vi "Do.vi"(8 "error in (no error)":errorcluster, 10 "Actor in":refnum<class "Actor.lvclass">, 11 "Configure Arbitrary Sequence [SEQ] Msg":refnum<class "Configure Arbitrary Sequence [SEQ] Msg.lvclass">) -> (0 "error out":errorcluster, 2 "Actor out":refnum<class "Actor.lvclass">)   [LabVIEW 2014, in "CS++Fgen.lvlib" / "Configure Arbitrary Sequence [SEQ] Msg.lvclass"]
doc: "This VI delivers the message to the actor by calling the appropriate method(s) on the actor."
uses:
  Configure Arbitrary Sequence [SEQ] Msg.lvclass
  <vilib>/ActorFramework/Actor/Actor.lvclass
  CS++Fgen/CS++Fgen.lvclass
  Configure Arbitrary Sequence [SEQ].ctl
  CSPP_Core/Actors/CS++PVMonitor Messages/CS++PVUpdate Msg/CS++PVUpdate Msg.lvclass/CS++PVUpdate Msg.ctl
  CSPP_Core/Classes/CS++ProcessVariables/ProcessVariable/PV.lvclass/PV.ctl
  Configure Arbitrary Sequence [SEQ] Msg.lvclass/Configure Arbitrary Sequence [SEQ] Msg.ctl
  CSPP_Core/Classes/CS++ProcessVariables/ProcessVariable/PV.lvclass
  CSPP_Core/Actors/CS++PVMonitor Messages/CS++PVUpdate Msg/CS++PVUpdate Msg.lvclass
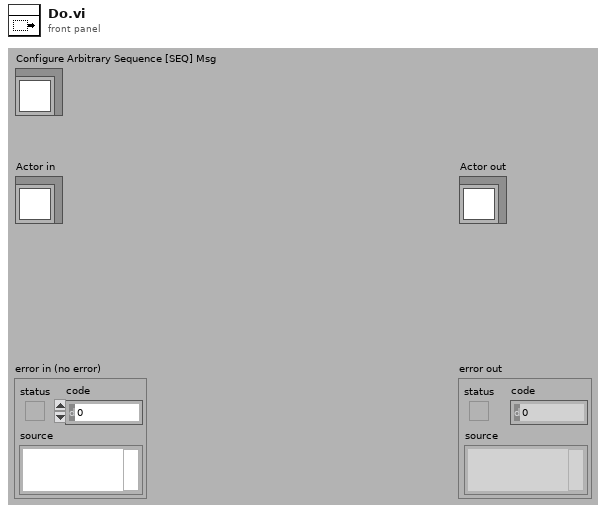
[diagram p1: front panel]
types:
  T1 = typedef "CS++Fgen.lvlib/Configure Arbitrary Sequence [SEQ] Msg.lvclass/Configure Arbitrary Sequence [SEQ].ctl" = cluster{"channel name (\"CHANNEL1\")":string, "offset (0.00 V)":dbl[unit], "gain (1.00)":dbl, "sequence handle (0)":i32}
  T2 = cluster{"channel name (\"CHANNEL1\")":string, "offset (0.00 V)":dbl[unit], "gain (1.00)":dbl, "sequence handle (0)":i32}
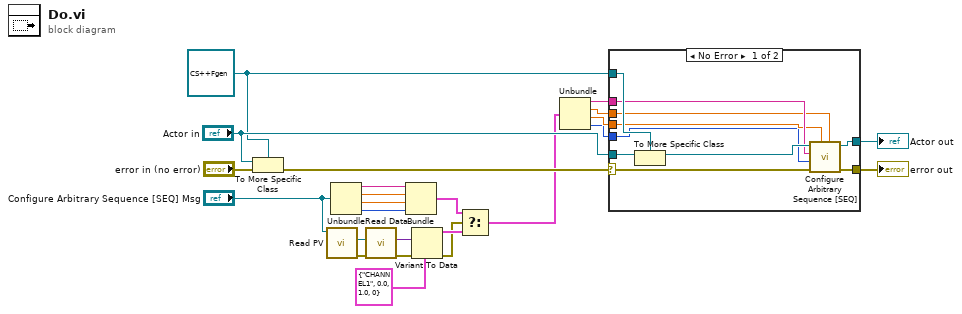
[diagram p0: block diagram]
diagram:
  w19 = refnum<class "CS++Fgen.lvclass"> refnum ("Actor in")
  n1 = To More Specific Class(target class=w19, reference="Actor in", error in="error in (no error)") -> (error out=w23:errorcluster)  [unwired: 1 out]
  n2 = call "Read PV.vi"("CS++PVUpdate Msg in"="Configure Arbitrary Sequence [SEQ] Msg") -> ("error out"=w2:errorcluster, "PV"=w14:refnum<class "PV.lvclass">)  [unwired: 8 in, 1 out]
  n3 = Unbundle("Configure Arbitrary Sequence [SEQ] Msg") -> (w9:string, w11:dbl[unit], w7:dbl, w6:i32)
  n4 = call "Read Data.vi"("error in (no error)"=w2, "PV in"=w14) -> ("error out"=w3:errorcluster, "Data"=w12:variant)  [unwired: 7 in, 1 out]
  n5 = Bundle("channel name (\"CHANNEL1\")"=w9, "offset (0.00 V)"=w11, "gain (1.00)"=w7, "sequence handle (0)"=w6) -> (w10:T2)  [unwired: 1 in]
  n6 = Variant To Data(error in=w3, type=T1 {"channel name (\"CHANNEL1\")"="CHANNEL1", "offset (0.00 V)"=0.0, "gain (1.00)"=1.0, "sequence handle (0)"=0} ("Cluster of class private data"), Variant=w12) -> (data=w13:T1, error out=w4:errorcluster)
  n7 = Select(t=w10, s=w4, f=w13) -> (s? t:f=w5:T1)
  n8 = Unbundle(w5) -> ("channel name (\"CHANNEL1\")"=w18:string, "offset (0.00 V)"=w17:dbl[unit], "gain (1.00)"=w16:dbl, "sequence handle (0)"=w15:i32)
  n9 = case shown="No Error" w23 {
    selector: w23 -> [w32 w36]
    tunnel: [w34 w36] -> w22
    tunnel: [w33 w35] -> w21
    tunnel: "Actor in" -> [w31 w35]
    tunnel: w19 -> [w30 _]
    tunnel: w18 -> [w28 _]
    tunnel: w17 -> [w27 _]
    tunnel: w16 -> [w26 _]
    tunnel: w15 -> [w25 _]
    frame No Error {
      n10 = To More Specific Class(target class=w30, reference=w31) -> (specific class reference=w29:refnum<class "CS++Fgen.lvclass">)  [unwired: 1 in, 1 out]
      n11 = call "Configure Arbitrary Sequence [SEQ].vi"("offset (0.00 V)"=w27, "gain (1.00)"=w26, "error in (no error)"=w32, "sequence handle (0)"=w25, "channel name (\"CHANNEL1\")"=w28, "CS++Fgen in"=w29) -> ("error out"=w34:errorcluster, "CS++Fgen out"=w33:refnum<class "CS++Fgen.lvclass">)  [unwired: 4 in]
    }
    frame Error {
      # "If type check fails, pass the original object out again."
    }
  }
  "error out" <- w22
  "Actor out" <- w21
